vi "Convert Digital to Analog Waveform Multi Channel.vi"(6 "Channels index":i32[](array[numeric]), 8 "full scale range":dbl=10.0 format="%#_13g", 9 "Number of samples":u32, 10 "Sample rate":dbl, 11 "Digital Waveform":u32[](array[numeric])) -> (3 "Waveforms":waveform(dbl)[](array[waveform]))   [LabVIEW 2021]
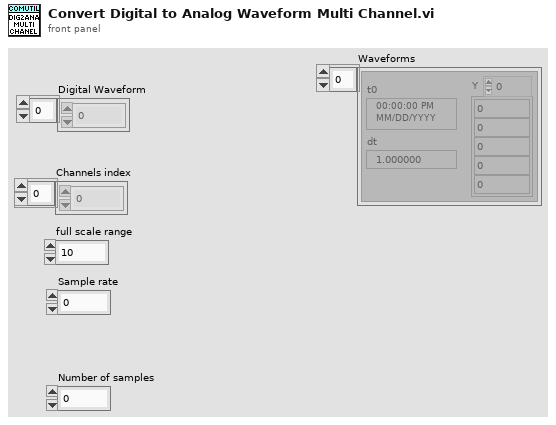
[diagram p1: front panel]
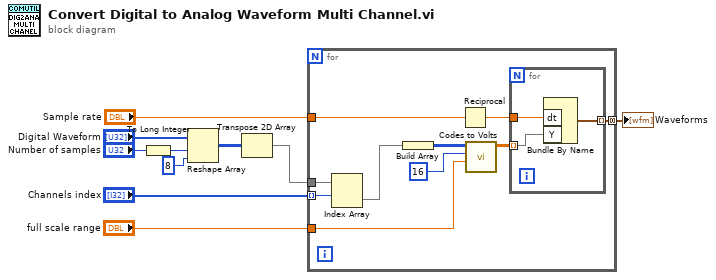
[diagram p0: block diagram]
diagram:
  n1 = To Long Integer(number="Number of samples") -> (32bit integer=w10:i32)
  n2 = Reshape Array("Digital Waveform", w10, 8 ("dimension size")) -> (w7:u32[][])
  n3 = Transpose 2D Array(2D array=w7) -> (transposed array=w3:u32[][])
  n4 = for {
    tunnel: "Sample rate" -> [w20]
    tunnel: [w16] -> w4 mode=concatenating
    tunnel: w3 -> [w15]
    tunnel: "Channels index" -> [w13] mode=indexing
    tunnel: "full scale range" -> [w11]
    n5 = Index Array(array=w15, index (row)=w13) -> (element=w14:u32[])  [unwired: 1 in]
    n6 = Build Array(w14) -> (w12:u32[][])
    n7 = Reciprocal(x=w20) -> (1/x=w19:dbl)
    n8 = call "Codes to Volts.vi"("full scale range"=w11, "number of bits"=16, "data"=w12) -> ("scaled data"=w17:dbl[][])  [unwired: 7 in, 1 out]
    n9 = for {
      tunnel: w19 -> [w23]
      tunnel: w17 -> [w22] mode=indexing
      tunnel: [w21] -> w16 mode=indexing
      n10 = Bundle By Name("dt"=w23, "Y"=w22) -> (w21:waveform(dbl))  [unwired: 1 in]
    }
  }
  "Waveforms" <- w4
